vi "FG Angle Mode.vi"(7 "action (read)":enum16{"read", "write"}(ring), 8 "error in (no error)":errorcluster, 11 "angle mode in":T1=1 items=["Degrees", "Radians"]) -> (0 "error out":errorcluster, 3 "angle mode out":T1=1 items=["Degrees", "Radians"])   [LabVIEW 2017, in "NI_Robotics_Configure Steering Frame.lvlib"]
uses:
  <vilib>/robotics/Dialog/Configure Steering Frame/NI_Robotics_Configure Steering Frame.lvlib
  <vilib>/robotics/Dialog/Configure Steering Frame/Angle Mode.ctl
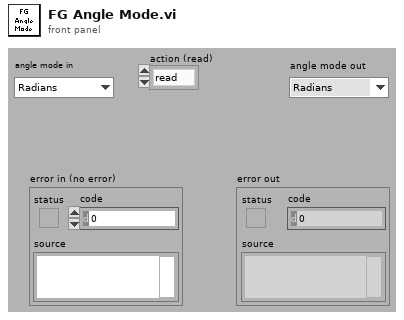
[diagram p1: front panel]
types:
  T1 = typedef "NI_Robotics_Configure Steering Frame.lvlib/Angle Mode.ctl" = u16
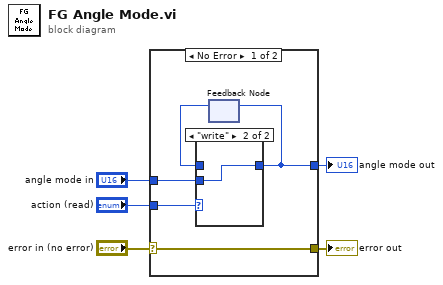
[diagram p0: block diagram]
diagram:
  n1 = case shown="No Error" "error in (no error)" {
    selector: "error in (no error)" -> [w10 w13]
    tunnel: [w10 w13] -> w4
    tunnel: "action (read)" -> [w9 _]
    tunnel: "angle mode in" -> [w8 _]
    tunnel: [w7 _] -> w1
    frame No Error {
      n2 = feedback #1() -> (w6:T1)  [unwired: 1 in]
      n3 = case shown="\"write\"" w9 {
        tunnel: w8 -> [_ w12]
        tunnel: [w11 w12] -> w7
        tunnel: w6 -> [w11 _]
        frame "read", Default {
        }
        frame "write" {
        }
      }
      n4 = feedback-in #1(w7) -> ()
    }
    frame Error {
    }
  }
  "angle mode out" <- w1
  "error out" <- w4
